vi "useClassInVariant.vi"() -> (3 "variant":variant)   [LabVIEW 2010]
uses:
  ClassDefinitions/SimpleClassWithProperties/myClass.lvclass
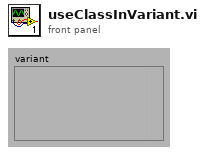
[diagram p1: front panel]
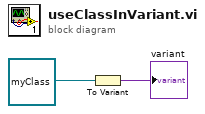
[diagram p0: block diagram]
diagram:
  n1 = To Variant(anything=refnum<class "myClass.lvclass"> refnum ("myClass.lvclass")) -> (Variant=→"variant":variant)
